vi "Material-Application-ProjectItemTypes.vi"(11 "error in":errorcluster) -> (4 "Deployments Root GUID":string="{BEECCB5A-0000-4BC9-973B-EDB26338DA05}", 6 "Application Deployment GUID":string="{BEECCB5A-0001-4BC9-973B-EDB26338DA05}", 8 "App Component Deployment GUID":string="{BEECCB5A-0002-4BC9-973B-EDB26338DA05}", 10 "Add New GUID":string="{BEECCB5A-0002-4BC9-973B-EDB26338DA05}", 15 "error out":errorcluster)   [LabVIEW 2013]
panel:
  # "Inputs"
  # "Outputs"
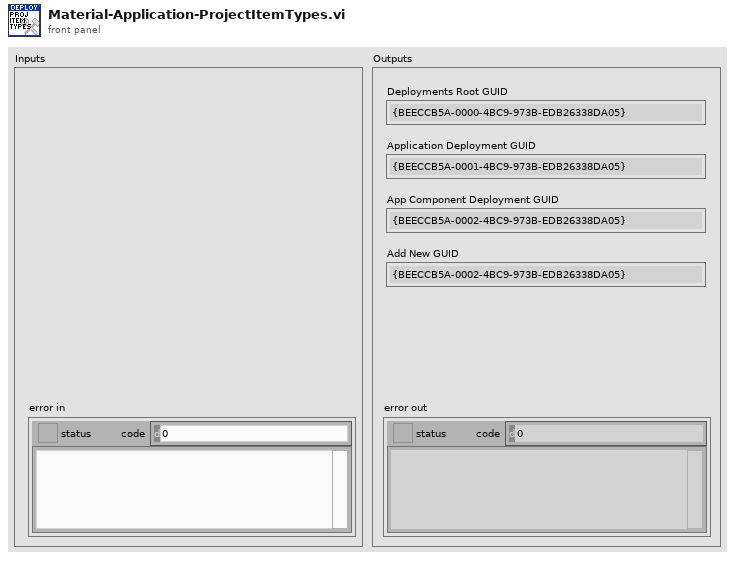
[diagram p1: front panel]
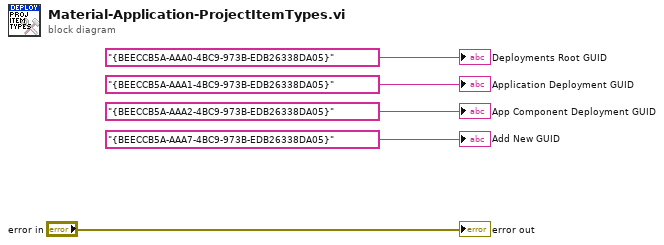
[diagram p0: block diagram]
diagram:
  "error out" <- "error in"
  "Application Deployment GUID" <- "{BEECCB5A-AAA1-4BC9-973B-EDB26338DA05}"
  "Deployments Root GUID" <- "{BEECCB5A-AAA0-4BC9-973B-EDB26338DA05}"
  "App Component Deployment GUID" <- "{BEECCB5A-AAA2-4BC9-973B-EDB26338DA05}"
  "Add New GUID" <- "{BEECCB5A-AAA7-4BC9-973B-EDB26338DA05}"
